vi "Teleop.vi"(10 "Match Info":T1={"Autonomous Elapsed Seconds"=0.0, "TeleOp Elapsed Seconds"=0.0, "Disabled Elapsed Seconds"=0.0, "Visited Autonomous"=FALSE, "Visited TeleOp"=FALSE, "Visited Disabled"=FALSE, "Autonomous Settings"={"Autonomous Style"=enum."Independent", "VI Refnum"=refnum}}, 11 "Call Context":T2) -> ()   [LabVIEW 2015]
doc: "This VI is called for each enabled TeleOp packet received from the DS. It is typically used to read from joysticks and other inputs and update I/O or setpoints for timed control loops. It should complete and return within 20 milliseconds or risk missing DS packets."
uses:
  <vilib>/Rock Robotics/WPI/DriverStation/WPI_DriverStationDerivedRobotMode.ctl
  <vilib>/Rock Robotics/WPI/DriverStation/WPI_DriverStationMatch Info.ctl
  Support Code/Team900-VIs/Logitech/F510/F510-X.vi
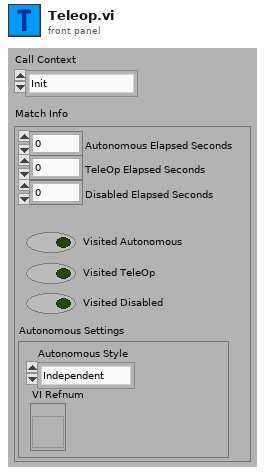
[diagram p1: front panel]
types:
  T1 = typedef "WPI_DriverStationMatch Info.ctl" = cluster{"Autonomous Elapsed Seconds":dbl, "TeleOp Elapsed Seconds":dbl, "Disabled Elapsed Seconds":dbl, "Visited Autonomous":bool, "Visited TeleOp":bool, "Visited Disabled":bool, "Autonomous Settings":cluster{"Autonomous Style":enum16{"Iterative", "Independent"}, "VI Refnum":refnum<vi>}}
  T2 = typedef "WPI_DriverStationDerivedRobotMode.ctl" = enum16{"Init", "Execute", "Stop"}
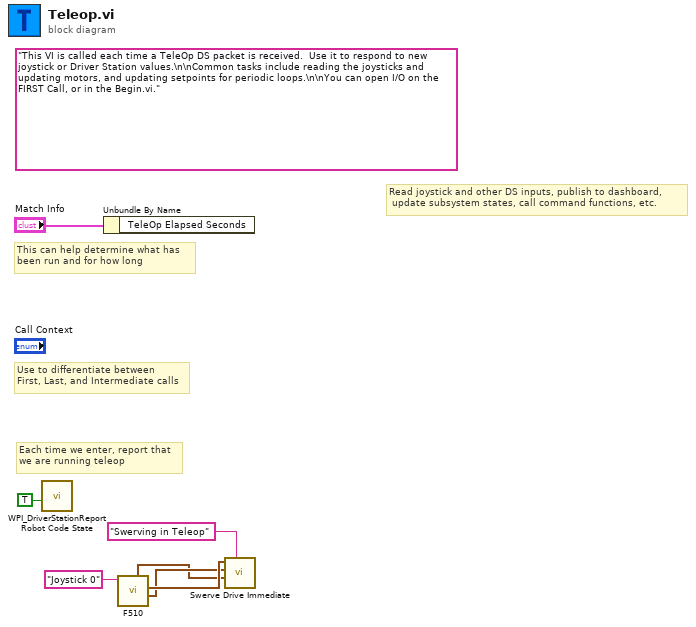
[diagram p0: block diagram]
diagram:
  (unwired) "This VI is called each time a TeleOp DS packet is received.  Use it to respond to new joystick or Driver Station values.\n\nCommon tasks include reading the joysticks and updating motors, and updating setpoints for periodic loops.\n\nYou can open I/O on the FIRST Call, or in the Begin.vi."
  # "Read joystick and other DS inputs, publish to dashboard,\n update subsystem states, call command functions, etc."
  # "Each time we enter, report that\nwe are running teleop"
  # "Use to differentiate between\nFirst, Last, and Intermediate calls"
  # "This can help determine what has\nbeen run and for how long"
  n1 = call <vilib>:"WPI_DriverStationReport Robot Code State.vi"("TeleOp"=TRUE ("Autonomous")) -> ()  [unwired: 10 in, 1 out]
  n2 = Unbundle By Name("Match Info") -> ()  [unwired: 1 out]
  n3 = call-poly "F510.vi"("refnum name"="Joystick 0") -> ("Right Stick"=w2:cluster{"X":dbl, "Y":dbl}, "Left Stick"=w3:cluster{"X":dbl, "Y":dbl}, "Triggers"=w1:cluster{"Left":dbl, "Right":dbl})  [unwired: 4 in, 4 out]
  n4 = call "Swerve Drive Immediate.vi"("Description"="Swerving in Teleop", "Trigger Axes"=w1, "Face Joystick Axes"=w2, "Strafe Joystick Axes"=w3) -> ()  [unwired: 7 in, 1 out]
